vi "tm_getparameterlist_40.vi"(8 "error in (no error)":errorcluster, 11 "Handle in":u32) -> (0 "error out":errorcluster, 2 "Function List":T1(array[cluster]), 3 "Handle out":u32)   [LabVIEW 2023]
uses:
  tmcamcon.dll
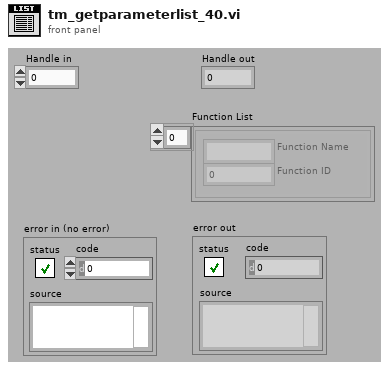
[diagram p1: front panel]
types:
  T1 = cluster{"Function Name":string, "Function ID":u32}[]
  T2 = cluster{"Property Name":string, "Property ID":i32}[]
  T3 = cluster{"Property Name":string, "Property ID":i32}
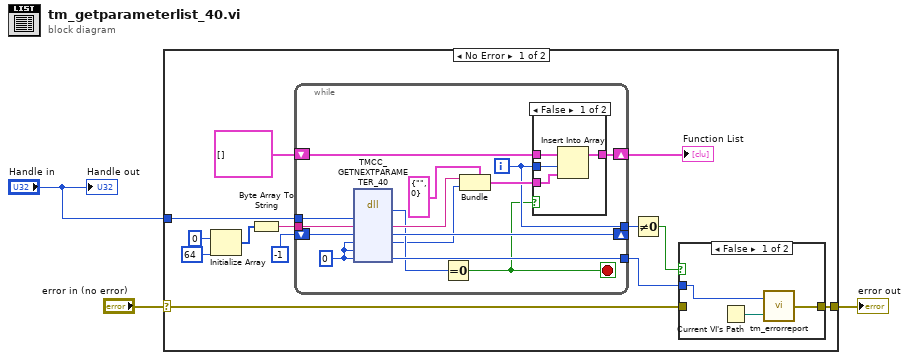
[diagram p0: block diagram]
diagram:
  n1 = case shown="No Error" "error in (no error)" {
    selector: "error in (no error)" -> [w8 w41]
    tunnel: [w5 w41] -> w2
    tunnel: "Handle in" -> [w9 _]
    frame No Error {
      n2 = Initialize Array(u8 0 ("element"), 64 ("dimension size")) -> (w10:u8[])
      n3 = Byte Array To String(unsigned byte array=w10) -> (string=w13:string)
      n4 = while {
        shift-right: [w34] -> w15
        shift-left: T2 [] ("Array") -> [w35]
        tunnel: [w30] -> w7
        tunnel: [w28] -> w14
        tunnel: w13 -> [w27]
        tunnel: w9 -> [w26]
        shift-right: [w29] -> _
        shift-left: -1 ("func_num") -> [w31]
        i -> [w28]
        stop <- w24 stop-if-true
        w21 = 0 ("option")
        n5 = dll-call lib="tmcamcon.dll" fn="TMCC_GETNEXTPARAMETER_40"("HDCAM"=w26, "name"=w27, "func_num"=w31, "func_id"=w21, "option"=w21, "Erval"=w21) -> ("return type"=w23:u32, "name"=w32:string, "func_num"=w29:i32, "func_id"=w22:i32, "Erval"=w30:i32)  [unwired: 5 in, 2 out]
        n6 = Equal To 0?(x=w23) -> (x = 0?=w24:bool)
        n7 = Bundle(cluster=T3 {"Property Name"="", "Property ID"=0} ("new element/subarray"), "Property Name"=w32, "Property ID"=w22) -> (w33:T3)
        n8 = case shown="False" w24 {
          tunnel: w35 -> [w39 w40]
          tunnel: [w38 w40] -> w34
          tunnel: w28 -> [w37 _]
          tunnel: w33 -> [w36 _]
          frame False {
            n9 = Insert Into Array(array=w39, index=w37, new element=w36) -> (w38:T2)
          }
          frame True {
          }
        }
      }
      "Function List" <- w15
      n10 = Not Equal To 0?(x=w14) -> (x != 0?=w6:bool)
      n11 = case shown="False" w6 {
        tunnel: w8 -> [_ w20]
        tunnel: [w18 w20] -> w5
        tunnel: w7 -> [w17 _]
        frame False {
          n12 = Current VI's Path() -> (path=w19:path)
          n13 = call "tm_errorreport.vi"("Source"=w19, "Error"=w17) -> ("error out"=w18:errorcluster)
        }
        frame True {
        }
      }
    }
    frame Error {
    }
  }
  "error out" <- w2
  "Handle out" <- "Handle in"
